vi "AlarmReset.vi"(9 "HighSpeedEServer":refnum<k24>, 11 "error in (no error)":errorcluster) -> (3 "error out":errorcluster)   [LabVIEW 2014, in "UnderAutomation.Yaskawa.lvlib"]
uses:
  UnderAutomation.Yaskawa.lvlib
  C:/Users/fg/Documents/Yaskawa.vi/LabVIEW_2024/UnderAutomation.Yaskawa/lib/UnderAutomation.Yaskawa.dll
  LabVIEW_2024/UnderAutomation.Yaskawa/lib/UnderAutomation.Yaskawa.dll
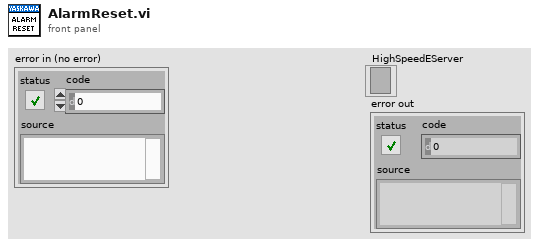
[diagram p1: front panel]
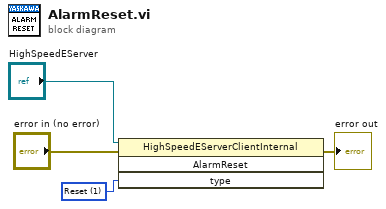
[diagram p0: block diagram]
diagram:
  w2 = 1 items=["Reset"=1, "Cancel"=2] ("type")
  n1 = invoke class="HighSpeedEServerClientInternal" method="AlarmReset"(reference="HighSpeedEServer", error in="error in (no error)", "type"=w2) -> (error out=→"error out":errorcluster)  [unwired: 1 in, 3 out]
